vi "Send scripted data to robot.vi"(10 "Programs":string[](array[string]), 11 "Program Name":string[](array[string])) -> ()   [LabVIEW 2013]
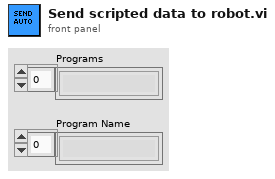
[diagram p1: front panel]
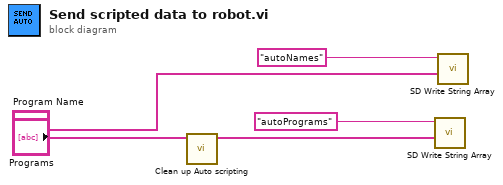
[diagram p0: block diagram]
diagram:
  n1 = call "Clean up Auto scripting.vi"("Programs"="Programs") -> ("Array"=w1:string[])  [unwired: 10 in]
  n2 = call <vilib>:"SD Write String Array.vi"("String Array"=w1, "Name"="autoPrograms") -> ()  [unwired: 8 in, 2 out]
  n3 = call <vilib>:"SD Write String Array.vi"("String Array"="Program Name", "Name"="autoNames") -> ()  [unwired: 8 in, 2 out]
